vi "XDOUT.VI"() -> ()   [LabVIEW 2010]
panel:
  out "Binary representation of \"Value\"":u32 format="%.0b"
  out "Decimal representation of \"Value\"":u32
  in  "Stop":bool
  out "DOut ErrMsg":string="No error has occurred"
  out "DConfigPort ErrMsg":string
  in  "Value":T1
  in  "BoardNum":u32
  in  "PortNum":i32(ring)=1 items=["AUXPORT", "FIRSTPORTA", "FIRSTPORTB", "FIRSTPORTCL", "FIRSTPORTCH", "SECONDPORTA", "SECONDPORTB", "SECONDPORTCL", "SECONDPORTCH", "THIRDPORTA", "THIRDPORTB", "THIRDPORTCL", "THIRDPORTCH", "FOURTHPORTA", "FOURTHPORTB", "FOURTHPORTCL", "FOURTHPORTCH", "FIFTHPORTA", "FIFTHPORTB", "FIFTHPORTCL", "FIFTHPORTCH", "SIXTHPORTA", "SIXTHPORTB", "SIXTHPORTCL", "SIXTHPORTCH", "SEVENTHPORTA", "SEVENTHPORTB", "SEVENTHPORTCL", "SEVENTHPORTCH", "EIGTHPORTA", "EIGHTHPORTB", "EIGHTHPORTCL", "EIGHTHPORTCH"]
  out "?":u32 format="%.0x"
  # "Demo for the DOut.VI and DCfgPort.VI corresponding to the Universal Library functions  cbDOut() and cbDConfigPort().\n\nConfigures the digital port and outputs the value to the port."
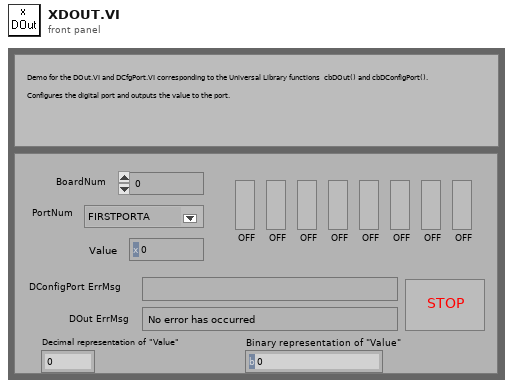
[diagram p1: front panel]
types:
  T1 = cluster{"Boolean":bool, "Boolean 2":bool, "Boolean 3":bool, "Boolean 4":bool, "Boolean 5":bool, "Boolean 6":bool, "Boolean 7":bool, "Boolean 8":bool}
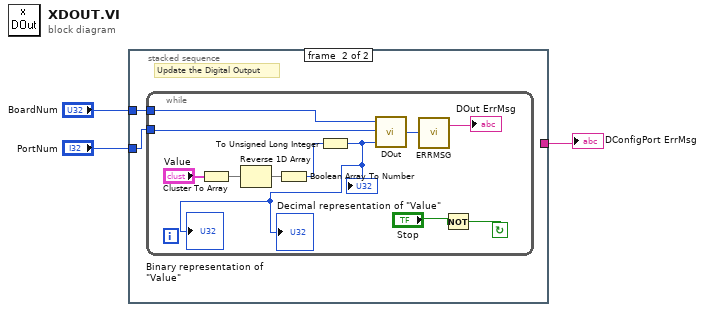
[diagram p0: block diagram]
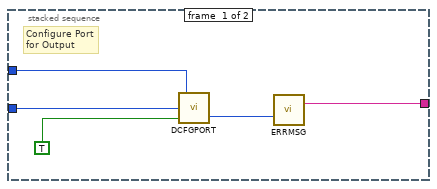
[diagram p2: hidden frame]
diagram:
  n1 = stacked-sequence {
    tunnel: [w8 _] -> w3
    tunnel: "BoardNum" -> [w5 w10]
    tunnel: "PortNum" -> [w4 w9]
    frame #0 {
      # "Configure Port \nfor Output"
      n2 = call "DCFGPORT.VI"("Direction"=TRUE, "PortNum"=w4, "BoardNum"=w5) -> ("ErrCode"=w7:i32)  [unwired: 1 out]
      n3 = call "ERRMSG.VI"("ErrCode"=w7) -> ("ErrMsg"=w8:string)  [unwired: 1 out]
    }
    frame #1 {
      # "Update the Digital Output"
      n4 = while {
        tunnel: w9 -> [w15]
        tunnel: w10 -> [w16]
        stop <- w17 continue-if-true
        n5 = Cluster To Array(cluster="Value") -> (array=w13:bool[])
        n6 = Reverse 1D Array(array=w13) -> (reversed array=w12:bool[])
        n7 = Boolean Array To Number(Boolean array=w12) -> (number=w14:u32)
        n8 = To Unsigned Long Integer(number=w14) -> (unsigned 32bit integer=w11:u32)
        "?" <- w11
        "Binary representation of \"Value\"" <- w11
        "Decimal representation of \"Value\"" <- w11
        n9 = call "DOut.VI"("DataValue"=w11, "PortNum"=w15, "BoardNum"=w16) -> ("ErrCode"=w20:i32)
        n10 = call "ERRMSG.VI"("ErrCode"=w20) -> ("ErrMsg"=→"DOut ErrMsg":string)  [unwired: 1 out]
        n11 = Not(x="Stop") -> (.not. x?=w17:bool)
      }
    }
  }
  "DConfigPort ErrMsg" <- w3
